vi "writeToXML.vi"(8 "error in (no error)":errorcluster, 10 "ClassLabel":string, 11 "WavefrontTargetConfiguration in":refnum<class "WavefrontTargetConfiguration.lvclass">) -> (0 "error out":errorcluster, 2 "XML out":string, 3 "WavefrontTargetConfiguration out":refnum<class "WavefrontTargetConfiguration.lvclass">)   [LabVIEW 2014, in "TCSDataDefinitions.lvlib" / "TCSCommand.lvlib" / "TargetConfiguration.lvlib" / "WavefrontTargetConfiguration.lvclass"]
uses:
  WavefrontTargetConfiguration.lvclass
  TargetConfiguration/TargetConfiguration.lvclass
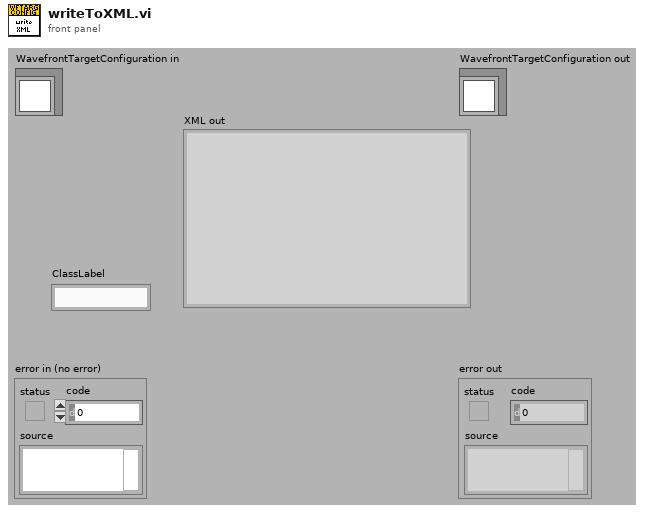
[diagram p1: front panel]
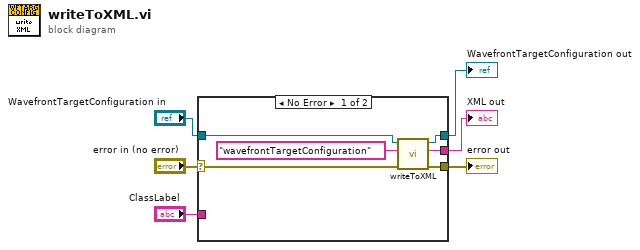
[diagram p0: block diagram]
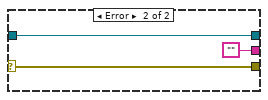
[diagram p2: hidden frame]
diagram:
  n1 = case shown="No Error" "error in (no error)" {
    selector: "error in (no error)" -> [w11 w15]
    tunnel: [w10 w15] -> w5
    tunnel: [w7 w14] -> w3
    tunnel: "WavefrontTargetConfiguration in" -> [w8 w14]
    tunnel: [w9 ""] -> w2
    tunnel: "ClassLabel" -> [_ _]
    frame No Error {
      n2 = call-parent "writeToXML.vi"("error in (no error)"=w11, "classLabel"="wavefrontTargetConfiguration", "TargetConfiguration in"=w8) -> ("error out"=w10:errorcluster, "XML out"=w9:string, "TargetConfiguration out"=w7:refnum<class "WavefrontTargetConfiguration.lvclass">)  [unwired: 6 in]
    }
    frame Error {
    }
  }
  "error out" <- w5
  "WavefrontTargetConfiguration out" <- w3
  "XML out" <- w2
